vi "Timer.vi"(1 "Timer Progress":refnum<vi>, 2 "Timer":dbl) -> ()   [LabVIEW 2010]
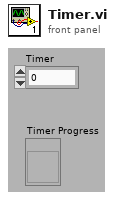
[diagram p1: front panel]
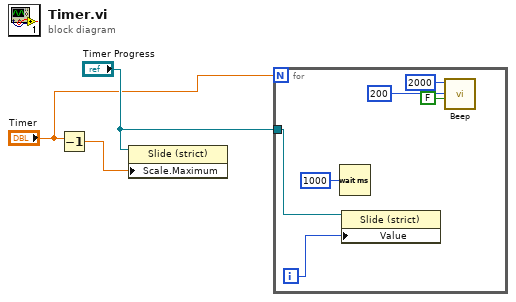
[diagram p0: block diagram]
diagram:
  n1 = Decrement(x="Timer") -> (x-1=w3:dbl)
  n2 = property class="Slide (strict)"(reference="Timer Progress", "Scale.Maximum"=w3) -> ()  [unwired: 1 in, 2 out]
  n3 = for {
    N: "Timer" -> [_]
    tunnel: "Timer Progress" -> [w8]
    i -> [w9]
    n4 = Wait (ms)(milliseconds to wait=u32 1000) -> ()  [unwired: 1 out]
    n5 = property class="Slide (strict)"(reference=w8, "Value"=w9) -> ()  [unwired: 1 in, 2 out]
    n6 = call <vilib>:"Beep.vi"("use system alert? (T)"=FALSE, "duration (msec)"=u32 200, "frequency (Hz)"=u32 2000) -> ()  [unwired: 9 in]
  }
